vi "On Change Start Stop Camera Preview.vi"(8 "error in (no error)":errorcluster, 10 "Value":bool, 11 "App in":refnum<class "App.lvclass">) -> (0 "error out":errorcluster, 3 "App out":refnum<class "App.lvclass">)   [LabVIEW 2020, in "AR Example.lvlib" / "App.lvclass"]
uses:
  App.lvclass
  App.lvclass/App.ctl
  UI/UI.lvclass
  Timeout Action.ctl
  g_ar_toolkit.common/Image Size (Integer).ctl
  g_ar_toolkit.capture/Stream/Camera Automatic Parameter Mode.ctl
  g_ar_toolkit.capture/Stream/Get Focus Parameter Info.vi
  g_ar_toolkit.capture/Stream/Set Automatic Focus Mode.vi.vi
  g_ar_toolkit.capture/Stream/Get Focus Parameter.vi
  g_ar_toolkit.capture/Stream/Camera Parameter Information.ctl
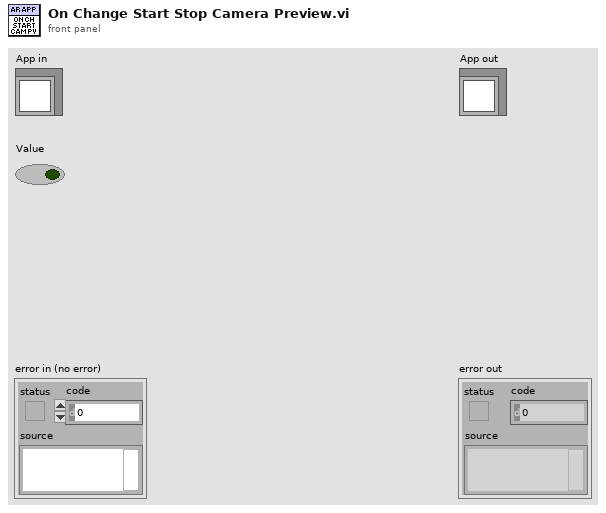
[diagram p1: front panel]
types:
  T1 = typedef "g_ar_toolkit.capture.lvlib/Stream.lvclass/Camera Parameter Information.ctl" = cluster{"Is Supported":bool, "Max":i32, "Min":i32, "Step":i32, "Default":i32}
  T2 = typedef "AR Example.lvlib/App.lvclass/Timeout Action.ctl" = enum16{"None", "Setup Camera Action", "Camera Calibration Action"}
  T3 = typedef "g_ar_toolkit.common.lvlib/Image Size (Integer).ctl" = cluster{"Width":u16, "Height":u16}
  T4 = typedef "g_ar_toolkit.capture.lvlib/Stream.lvclass/Camera Automatic Parameter Mode.ctl" = enum16{"Manual", "Automatic"}
  T5 = typedef "g_ar_toolkit.capture.lvlib/Stream.lvclass/Device Enumeration.ctl" = cluster{"Name":string, "Streams":set{T6}}
  T6 = typedef "g_ar_toolkit.capture.lvlib/Stream.lvclass/Stream Parameters.ctl" = cluster{"Width":u16, "Height":u16, "FPS":u8}
  T7 = typedef "g_ar_toolkit.image.lvlib/Image Draw Offset.ctl" = cluster{"Left":i16, "Top":i16}
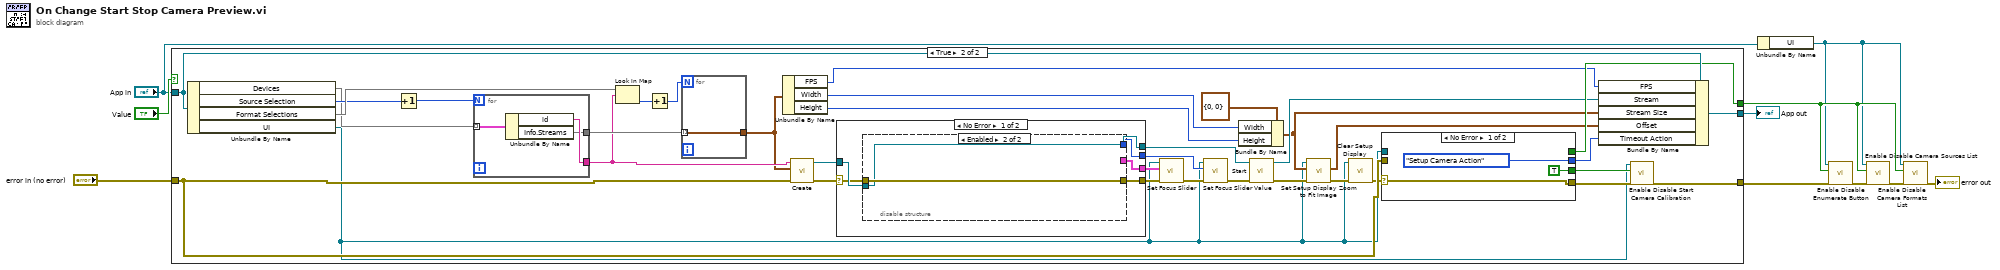
[diagram p0: block diagram]
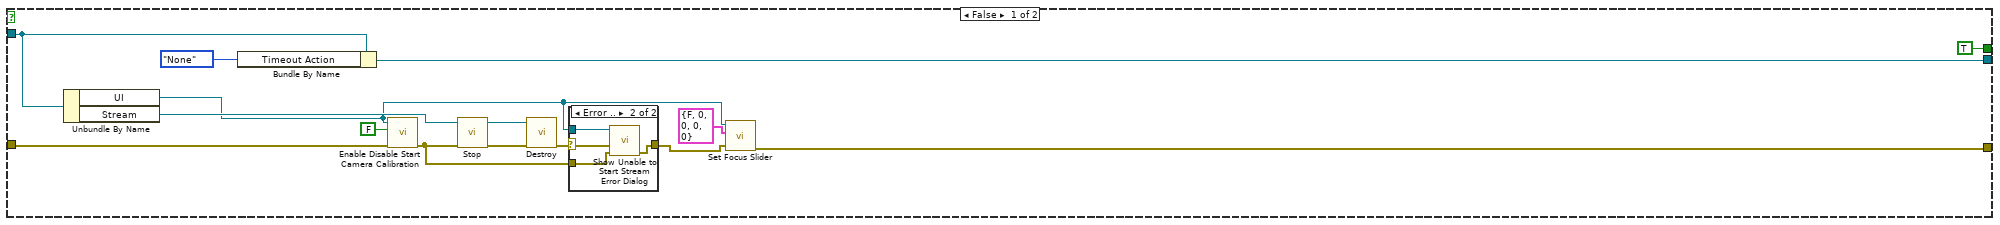
[diagram p2: hidden frame]
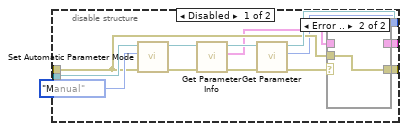
[diagram p4: hidden frame]
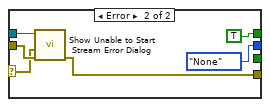
[diagram p7: hidden frame]
diagram:
  n1 = case shown="True" "Value" {
    tunnel: [w15 w33] -> w5
    tunnel: [w21 w58] -> w9
    tunnel: "App in" -> [w24 w66]
    tunnel: "error in (no error)" -> [w23 w56]
    tunnel: [TRUE w55] -> w6
    frame False {
      n2 = Unbundle By Name(w24) -> ("UI"=w12:refnum<class "UI.lvclass">, "Stream"=w19:refnum<class "Stream.lvclass">)
      n3 = Bundle By Name(cluster=w24, "Timeout Action"=Timeout_Action."None" ("Shared.Timeout Action")) -> (w21:refnum<class "App.lvclass">)
      n4 = call-dynamic "Enable Disable Start Camera Calibration.vi"("error in (no error)"=w23, "Enable?"=FALSE, "UI in"=w12) -> ("error out"=w13:errorcluster)  [unwired: 8 in]
      n5 = call "Stop.vi"("error in (no error)"=w13, "Stream in"=w19) -> ("error out"=w18:errorcluster, "Stream (Duplicate)"=w17:refnum<class "Stream.lvclass">)  [unwired: 8 in]
      n6 = call "Destroy.vi"("error in (no error)"=w18, "Stream in"=w17) -> ("error out"=w16:errorcluster)  [unwired: 9 in]
      n7 = case shown="Error .." w16 {
        selector: w16 -> [w26 w29]
        tunnel: w12 -> [_ w30]
        tunnel: w13 -> [_ w28]
        tunnel: [w26 w27] -> w22
        frame No Error {
        }
        frame Error {
          n8 = call-dynamic "Show Unable to Start Stream Error Dialog.vi"("error in (no error)"=w28, "Stream Start Error"=w29, "UI in"=w30) -> ("error out"=w27:errorcluster)  [unwired: 8 in]
        }
      }
      n9 = call "Set Focus Slider.vi"("error in (no error)"=w22, "Camera Parameter Information"=T1 {"Is Supported"=FALSE, "Max"=0, "Min"=0, "Step"=0, "Default"=0}, "UI in"=w12) -> ("error out"=w15:errorcluster)  [unwired: 8 in]
    }
    frame True {
      n10 = Unbundle By Name(w66) -> ("Devices"=w60:map{string, T5}, "Source Selection"=w62:i32, "Format Selections"=w65:map{string, i32}, "UI"=w31:refnum<class "UI.lvclass">)
      n11 = Increment(x=w62) -> (x+1=w61:i32)
      n12 = for {
        N: w61 -> [_]
        tunnel: w60 -> [w104] mode=indexing
        tunnel: [w103] -> w45
        tunnel: [w102] -> w59
        n13 = Unbundle By Name(w104) -> ("id"=w103:string, "Info.Streams"=w102:set{T6})
      }
      n14 = Look In Map(map=w65, key=w45) -> (value=w64:i32)  [unwired: 1 in, 1 out]
      n15 = Increment(x=w64) -> (x+1=w63:i32)
      n16 = for {
        N: w63 -> [_]
        tunnel: w59 -> [w105] mode=indexing
        tunnel: [w105] -> w43
      }
      n17 = Unbundle By Name(w43) -> ("FPS"=w46:u8, "Width"=w53:u16, "Height"=w52:u16)
      n18 = call "Create.vi"("error in (no error)"=w56, "Desired Stream Parameters"=w43, "Device ID"=w45) -> ("error out"=w40:errorcluster, "New Stream"=w41:refnum<class "Stream.lvclass">)  [unwired: 7 in]
      n19 = case shown="No Error" w40 {
        selector: w40 -> [w70 w92]
        tunnel: [w69 w92] -> w39
        tunnel: [w71 w91] -> w42
        tunnel: w41 -> [w72 w91]
        tunnel: [w68 _] -> w37
        tunnel: [w67 _] -> w35
        frame No Error {
          n20 = disable-structure shown="Enabled" {
            disable-tunnel: w72 -> [w84 w89]
            disable-tunnel: [w79 w89] -> w71
            disable-tunnel: w70 -> [w77 w90]
            disable-tunnel: [w76 w90] -> w69
            disable-tunnel: [w74 _] -> w68
            disable-tunnel: [w73 _] -> w67
            frame Disabled {
              n21 = call-poly "Set Automatic Parameter Mode.vi"("error in (no error)"=w77, "Automatic Parameter Mode"=Camera_Automatic_Parameter_Mode."Manual", "Stream in"=w84) -> ("error out"=w83:errorcluster, "Stream (Duplicate)"=w82:refnum<class "Stream.lvclass">)  [unwired: 7 in]
              n22 = call-poly "Get Parameter Info.vi"("error in (no error)"=w83, "Stream in"=w82) -> ("error out"=w81:errorcluster, "Info"=w75:T1, "Stream (Duplicate)"=w80:refnum<class "Stream.lvclass">)  [unwired: 7 in]
              n23 = call-poly "Get Parameter.vi"("error in (no error)"=w81, "Stream in"=w80) -> ("error out"=w78:errorcluster, "Value"=w73:i32, "Stream (Duplicate)"=w79:refnum<class "Stream.lvclass">)  [unwired: 7 in]
              n24 = case shown="Error .." w78 {
                selector: w78 -> [w87 _]
                tunnel: w77 -> [_ w88]
                tunnel: [w87 w88] -> w76
                tunnel: w75 -> [w86 _]
                tunnel: [w86 _] -> w74
                frame No Error {
                }
                frame Error {
                }
              }
            }
            frame Enabled {
            }
          }
        }
        frame Error {
        }
      }
      n25 = call "Set Focus Slider.vi"("error in (no error)"=w39, "Camera Parameter Information"=w37, "UI in"=w31) -> ("error out"=w38:errorcluster)  [unwired: 8 in]
      n26 = call "Set Focus Slider Value.vi"("error in (no error)"=w38, "Value"=w35, "UI in"=w31) -> ("error out"=w36:errorcluster)  [unwired: 8 in]
      n27 = Bundle By Name(cluster=T3 {"Width"=0, "Height"=0} ("Size"), "Width"=w53, "Height"=w52) -> (w34:T3)
      n28 = call "Start.vi"("error in (no error)"=w36, "Stream in"=w42) -> ("error out"=w51:errorcluster, "Stream (Duplicate)"=w44:refnum<class "Stream.lvclass">)  [unwired: 8 in]
      n29 = call-dynamic "Set Setup Display Zoom to Fit Image.vi"("error in (no error)"=w51, "Size"=w34, "UI in"=w31) -> ("error out"=w50:errorcluster, "Offset"=w49:T7)  [unwired: 7 in]
      n30 = call-dynamic "Clear Setup Display.vi"("error in (no error)"=w50, "UI in"=w31) -> ("error out"=w47:errorcluster)  [unwired: 9 in]
      n31 = case shown="No Error" w47 {
        selector: w47 -> [w95 w99]
        tunnel: [w95 w100] -> w57
        tunnel: w56 -> [_ w101]
        tunnel: [Timeout_Action."Setup Camera Action" ("Shared.Timeout Action") Timeout_Action."None" ("Shared.Timeout Action")] -> w48
        tunnel: [_ TRUE] -> w55
        tunnel: w31 -> [_ w96]
        tunnel: [TRUE _] -> w32
        frame No Error {
        }
        frame Error {
          n32 = call-dynamic "Show Unable to Start Stream Error Dialog.vi"("error in (no error)"=w101, "Stream Start Error"=w99, "UI in"=w96) -> ("error out"=w100:errorcluster)  [unwired: 8 in]
        }
      }
      n33 = Bundle By Name(cluster=w66, "FPS"=w46, "Stream"=w44, "Stream Size"=w34, "Offset"=w49, "Timeout Action"=w48) -> (w58:refnum<class "App.lvclass">)
      n34 = call-dynamic "Enable Disable Start Camera Calibration.vi"("error in (no error)"=w57, "Enable?"=w32, "UI in"=w31) -> ("error out"=w33:errorcluster)  [unwired: 8 in]
    }
  }
  "App out" <- w9
  n35 = Unbundle By Name("App in") -> ("UI"=w1:refnum<class "UI.lvclass">)
  n36 = call-dynamic "Enable Disable Enumerate Button.vi"("error in (no error)"=w5, "Enable?"=w6, "UI in"=w1) -> ("error out"=w4:errorcluster)  [unwired: 8 in]
  n37 = call-dynamic "Enable Disable Camera Sources List.vi"("error in (no error)"=w4, "Enable?"=w6, "UI in"=w1) -> ("error out"=w3:errorcluster)  [unwired: 8 in]
  n38 = call-dynamic "Enable Disable Camera Formats List.vi"("error in (no error)"=w3, "Enable?"=w6, "UI in"=w1) -> ("error out"=→"error out":errorcluster)  [unwired: 8 in]
